vi "Initialise.vi"(6 "Tag Root":string, 8 "error in (no error)":errorcluster, 9 "Values":refnum<class "Abs_Type.lvclass">[](array[class]), 10 "Tags":string[](array[string]), 11 "Aggregator Bus in":refnum<class "Aggregator Bus.lvclass">) -> (0 "error out":errorcluster, 3 "Aggregator Bus out":refnum<class "Aggregator Bus.lvclass">)   [LabVIEW 2021, in "Aggregator Bus.lvclass"]
uses:
  Aggregator Bus.lvclass
  Aggregator Bus.lvclass/Aggregator Bus.ctl
  <vilib>/TSA/Abstract Data Classes/Abs_Types/Type/Abs_Type.lvclass
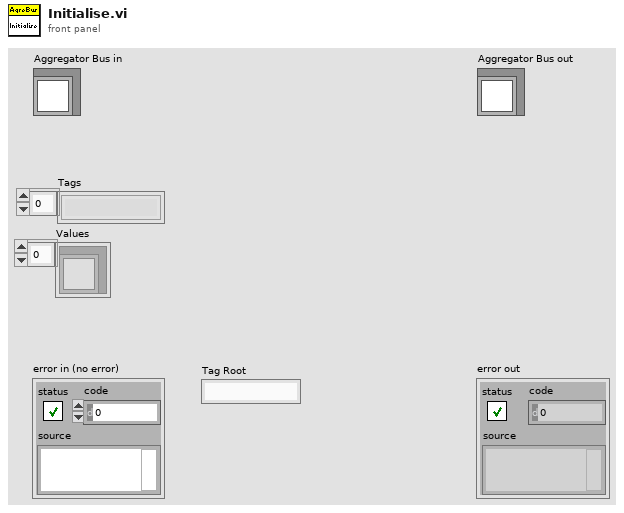
[diagram p1: front panel]
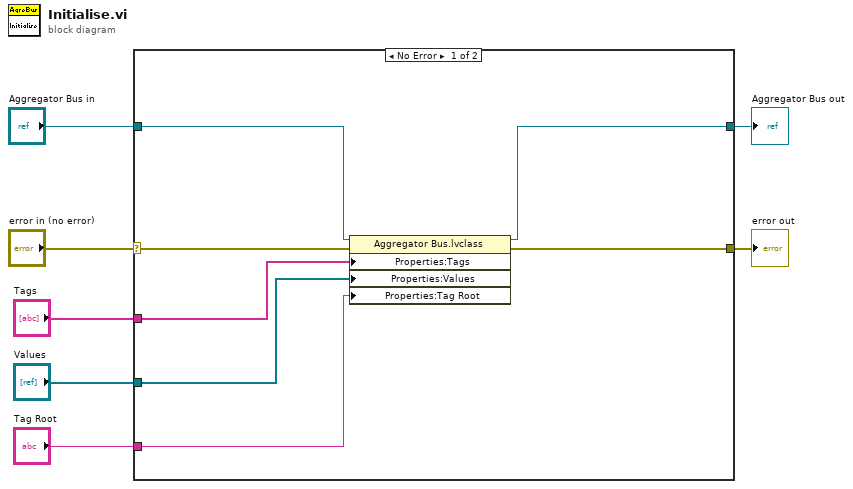
[diagram p0: block diagram]
diagram:
  n1 = case shown="No Error" "error in (no error)" {
    selector: "error in (no error)" -> [w13 w16]
    tunnel: [w11 w16] -> w6
    tunnel: [w12 w15] -> w4
    tunnel: "Aggregator Bus in" -> [w14 w15]
    tunnel: "Tags" -> [w10 _]
    tunnel: "Values" -> [w9 _]
    tunnel: "Tag Root" -> [w8 _]
    frame No Error {
      n2 = property class="Aggregator Bus.lvclass"(reference=w14, error in=w13, "Properties:Tags"=w10, "Properties:Values"=w9, "Properties:Tag Root"=w8) -> (reference out=w12:refnum<class "Aggregator Bus.lvclass">, error out=w11:errorcluster)
    }
    frame Error {
    }
  }
  "error out" <- w6
  "Aggregator Bus out" <- w4
